vi "Set Light RGB By Name.vi"(7 "Name":string, 8 "Error In":errorcluster, 10 "Color":u32(colorbox), 11 "Hue Config":T1) -> (0 "Error Out":errorcluster, 3 "Hue Config":T1)   [LabVIEW 2020]
uses:
  LMH-Hue.lvlib
  <vilib>/httpClient/ClientHandle.ctl
  <vilib>/httpClient/LabVIEWHTTPClient.lvlib
  Type Defs/Hue Ref.ctl
  Type Defs/Light Data.ctl
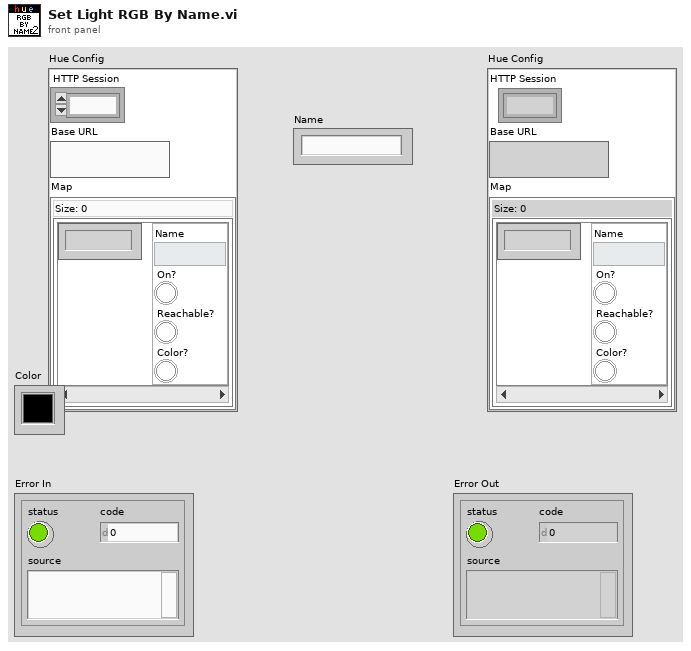
[diagram p1: front panel]
types:
  T1 = typedef "LMH-Hue.lvlib/Hue Ref.ctl" = cluster{"HTTP Session":T2, "Base URL":string, "Map":map{i32, T3}}
  T2 = typedef "LabVIEWHTTPClient.lvlib/ClientHandle.ctl" = refnum<k1>
  T3 = typedef "LMH-Hue.lvlib/Light Data.ctl" = cluster{"Name":string, "On?":bool, "Reachable?":bool, "Color?":bool}
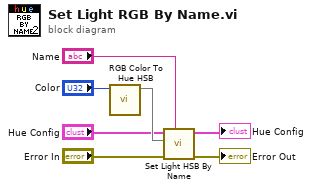
[diagram p0: block diagram]
diagram:
  n1 = call "RGB Color To Hue HSB.vi"(11:"Color") -> (3:w7)  [unwired: 9 in, 1 out]
  n2 = call "Set Light HSB By Name.vi"("Name"="Name", "Error In"="Error In", "HSB"=w7, "Hue Config"="Hue Config") -> ("Error Out"=→"Error Out":errorcluster, "Hue Config"=→"Hue Config":T1)  [unwired: 6 in]
